vi "sub-SetLanguageSel.vi"(11 "sel":i32) -> ()   [LabVIEW 2011]
uses:
  sub-Language global.vi
  <vilib>/Utility/config.llb/Write Key (I32).vi
  <vilib>/Utility/config.llb/NI_LVConfig.lvlib
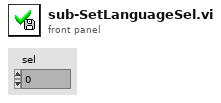
[diagram p1: front panel]
types:
  T1 = typedef "NI_LVConfig.lvlib/Config Data RefNum.ctl" = refnum<k1>
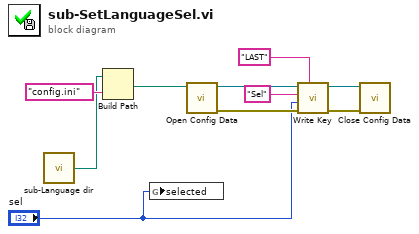
[diagram p0: block diagram]
diagram:
  n1 = call "sub-Language dir.vi"() -> ("folder"=w8:path)
  n2 = Build Path(base path=w8, name or relative path="config.ini" ("名称或相对路径")) -> (appended path=w9:path)
  n3 = global write "sub-Language global.vi" "selected"("sel") -> ()
  n4 = call <vilib>:"Open Config Data.vi"("configuration file path"=w9) -> ("error out"=w6:errorcluster, "refnum"=w7:T1)  [unwired: 8 in, 1 out]
  n5 = call-poly <vilib>:"Write Key.vi"("section"="LAST", "error in (no error)"=w6, "value"="sel", "key"="Sel", "refnum"=w7) -> ("error out"=w2:errorcluster, "refnum out"=w3:T1)  [unwired: 4 in, 1 out]
  n6 = call <vilib>:"Close Config Data.vi"("error in (no error)"=w2, "refnum"=w3) -> ()  [unwired: 8 in, 2 out]
